vi "Set gRPC ID.vi"(10 "gRPC ID":T1, 11 "OOP Server in":refnum<class "Template Server.lvclass">) -> (3 "OOP Server out":refnum<class "Template Server.lvclass">)   [LabVIEW 2019, in "Template Server.lvlib" / "Template Server.lvclass"]
uses:
  Template Server.lvclass
  gRPC interface/Server API/typeDefs/grpcId.ctl
  Template Server.lvclass/Template Server.ctl
  gRPC interface/gprc-lvsupport.lvlib
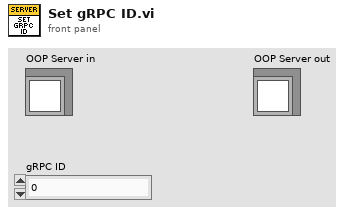
[diagram p1: front panel]
types:
  T1 = typedef "gprc-lvsupport.lvlib/grpcId.ctl" = u64
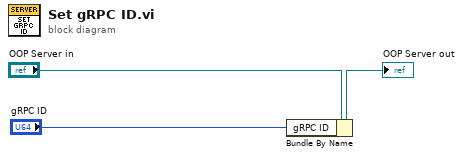
[diagram p0: block diagram]
diagram:
  n1 = Bundle By Name(cluster="OOP Server in", "gRPC ID"="gRPC ID") -> (→"OOP Server out":refnum<class "Template Server.lvclass">)
